vi "Security Level.vi"(8 "error in (no error)":errorcluster, 10 "Security Level (0: Off)":i32(ring) items=["Off", "Low", "High"], 11 "VISA resource name":refnum<visa-resource-name>) -> (0 "error out":errorcluster, 3 "VISA resource name out":refnum<visa-resource-name>)   [LabVIEW 2018, in "Agilent ENA Series.lvlib"]
doc: "Sets the security level.\n\nNotes:\n(1) This VI is not supported by the E5080A, E5070B/E5071B."
uses:
  Agilent ENA Series.lvlib
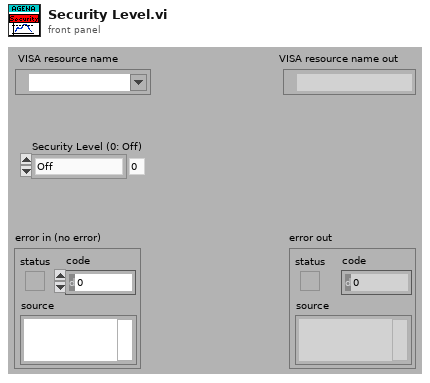
[diagram p1: front panel]
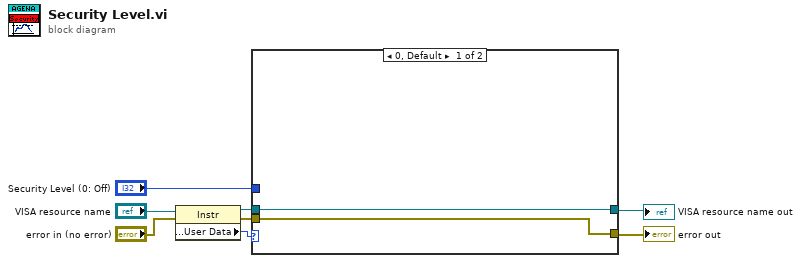
[diagram p0: block diagram]
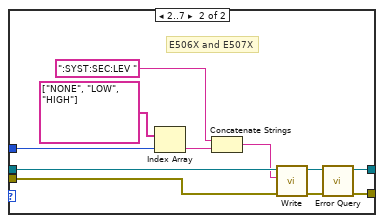
[diagram p2: hidden frame]
diagram:
  n1 = property class="Instr"(reference="VISA resource name", error in="error in (no error)") -> (reference out=w8:refnum<visa-resource-name>, error out=w7:errorcluster, "General Settings:User Data"=w6:u32)
  n2 = case shown="0, Default" w6 {
    tunnel: w8 -> [w10 w21]
    tunnel: w7 -> [w9 w20]
    tunnel: [w10 w12] -> w2
    tunnel: [w9 w11] -> w1
    tunnel: "Security Level (0: Off)" -> [_ w19]
    frame 0, Default {
    }
    frame 2..7 {
      # "E506X and E507X"
      n3 = Index Array(array=string[] ["NONE", "LOW", "HIGH"], index=w19) -> (element=w17:string)
      n4 = Concatenate Strings(":SYST:SEC:LEV ", w17) -> (w15:string)
      n5 = call "Write.vi"("error in (no error)"=w20, "String ()"=w15, "VISA resource name"=w21) -> ("error out"=w13:errorcluster, "VISA resource name out"=w14:refnum<visa-resource-name>)  [unwired: 6 in, 1 out]
      n6 = call "Error Query.vi"("error in (no error)"=w13, "VISA resource name"=w14) -> ("error out"=w11:errorcluster, "VISA resource name out"=w12:refnum<visa-resource-name>)  [unwired: 6 in, 2 out]
    }
  }
  "error out" <- w1
  "VISA resource name out" <- w2
